vi "Set Kinematic Parameters.vi"(8 "error in (no error)":errorcluster, 10 "kinematic parameters":T1, 11 "Finger in":refnum<class "Finger.lvclass">) -> (0 "error out":errorcluster, 3 "Finger out":refnum<class "Finger.lvclass">)   [LabVIEW 2011, in "Finger.lvclass"]
uses:
  Finger.lvclass
  Controls/Kinematic Parameters.ctl
  <vilib>/Analysis/Matrix/Datatypes/RealMatrix.ctl
  <vilib>/robotics/Kinematics/Link/Joint Type.ctl
  Controls/5-bar Side.ctl
  Finger.lvclass/Finger.ctl
  <vilib>/Analysis/Matrix/NI_Matrix.lvlib
  <vilib>/robotics/Kinematics/Link/NI_Robotics_Link.lvclass
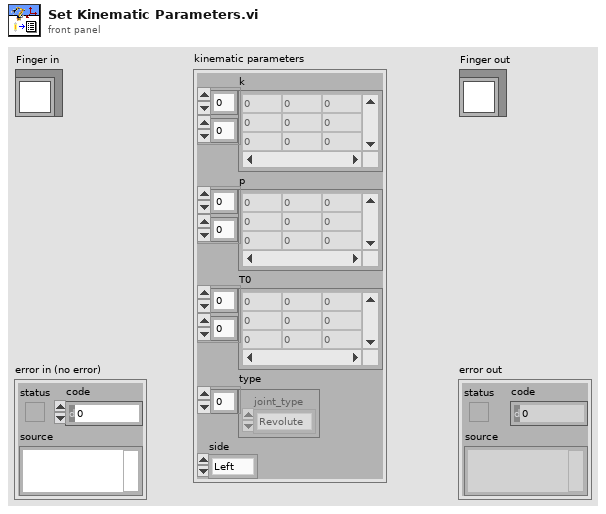
[diagram p1: front panel]
types:
  T1 = typedef "Kinematic Parameters.ctl" = cluster{"k":T2, "p":T2, "T0":T2, "type":T3[], "side":T4}
  T2 = typedef "NI_Matrix.lvlib/RealMatrix.ctl" = dbl[][]
  T3 = typedef "NI_Robotics_Link.lvclass/Joint Type.ctl" = enum16{"Revolute", "Prismatic"}
  T4 = typedef "5-bar Side.ctl" = enum16{"Left", "Right"}
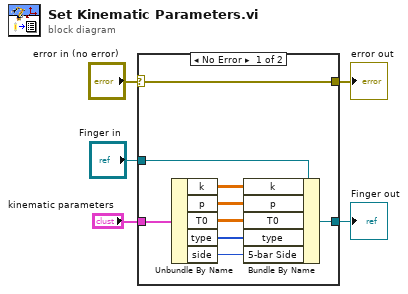
[diagram p0: block diagram]
diagram:
  n1 = case shown="No Error" "error in (no error)" {
    selector: "error in (no error)" -> [w14 w16]
    tunnel: [w14 w16] -> w4
    tunnel: [w12 w15] -> w2
    tunnel: "Finger in" -> [w13 w15]
    tunnel: "kinematic parameters" -> [w7 _]
    frame No Error {
      n2 = Unbundle By Name(w7) -> ("k"=w11:T2, "p"=w10:T2, "T0"=w9:T2, "type"=w8:T3[], "side"=w6:T4)
      n3 = Bundle By Name(cluster=w13, "k"=w11, "p"=w10, "T0"=w9, "type"=w8, "5-bar Side"=w6) -> (w12:refnum<class "Finger.lvclass">)
    }
    frame Error {
    }
  }
  "error out" <- w4
  "Finger out" <- w2
